vi "cls34401.vi"(1 "error in":errorcluster, 2 "VISA session 2":refnum<visa-resource-name>) -> (0 "error out":errorcluster)   [LabVIEW 2012]
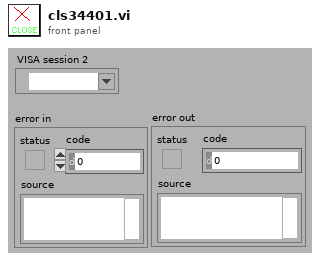
[diagram p1: front panel]
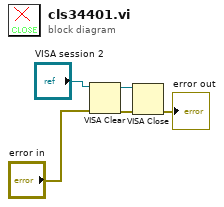
[diagram p0: block diagram]
diagram:
  n1 = VISA Clear(VISA resource name="VISA session 2", error in (no error)="error in") -> (VISA resource name out=w3:refnum<visa-resource-name>, error out=w5:errorcluster)
  n2 = VISA Close(VISA resource name=w3, error in (no error)=w5) -> (error out=→"error out":errorcluster)
